vi "Remove Vx from Project.vi"(11 "Project File":path=path "C:/Users/Steve/Documents/LabVIEW/DePuy test rig software new - Playing/DePuy test rig software.lvproj") -> ()   [LabVIEW 2015]
uses:
  Sub VIs/Rename Vx States.ctl
  <vilib>/Utility/file.llb/Write Delimited Spreadsheet (string).vi
  <vilib>/Utility/file.llb/Read Delimited Spreadsheet (string).vi
  <vilib>/LabVIEW Icon API/LabVIEW Icon API.lvlib
panel:
  out "Count":i32
  out "All VIs Count":i32
  in  "Edit ICONs":bool
  out "State":T1
  in  "Delete Originals":bool
  out "Rename Array":path[][](array[path])
  out "All VIs":path[](array[path])
  out "All VI Files":path
  in  "ReLink VIs":bool
  in  "Rename Files in Project":bool
  in  "Revert":bool
  in  "Rename Files":bool
  in  "Load Rename File":bool
  in  "Save Rename File":bool
  out "Rename Files":path
  in  "Read Project":bool
  in  "Stop":bool
  out "Selection Array":T2(array[cluster])
  in  "Ignore Folders":path[](array[path])=[path "C:/Users/Steve/Documents/LabVIEW/DePuy test rig software new - Playing/data", path "C:/Users/Steve/Documents/LabVIEW/DePuy test rig software new - Playing/DLLs", path "C:/Users/Steve/Documents/LabVIEW/DePuy test rig software new - Playing/sub vis/data", path "C:/Users/Steve/Documents/LabVIEW/DePuy test rig software new - Playing/sub vis/data old", path "C:/Users/Steve/Documents/LabVIEW/DePuy test rig software new - Playing/Mathcad Worksheets"]
  # "COMMIT Renamed Files\n    Change Missing to Deleted\n    Change Unknown to Added\n    All should show as Renamed"
  # "Cancel in ICON Editor to Stop"
  # "COMMIT Relinked Files"
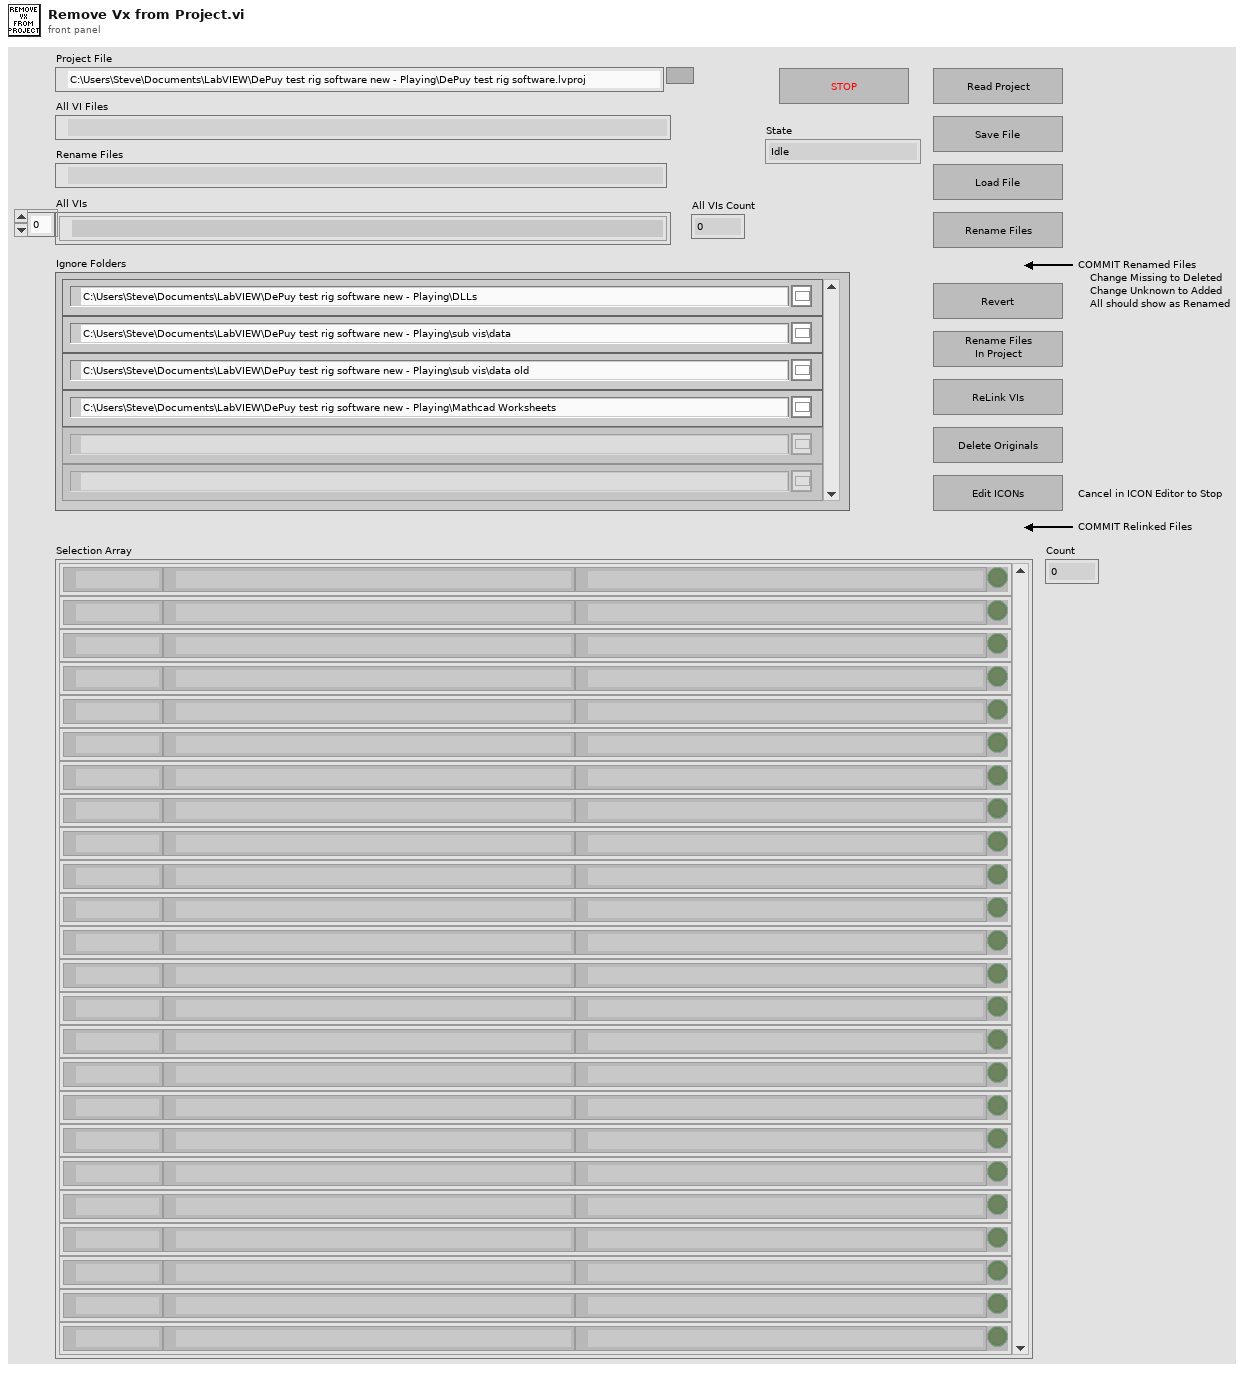
[diagram p1: front panel]
types:
  T1 = typedef "Rename Vx States.ctl" = enum16{"Idle", "Read Project", "Save File", "Load File", "Rename Files", "Revert", "Rename Files in Project", "Delete Originals", "Relink VIs", "Edit ICONs", "Exit"}
  T2 = cluster{"Original":path, "Name":path, "Rename":path, "Change":bool}[]
  T3 = cluster{"Original":path, "Name":path, "Rename":path, "Change":bool}
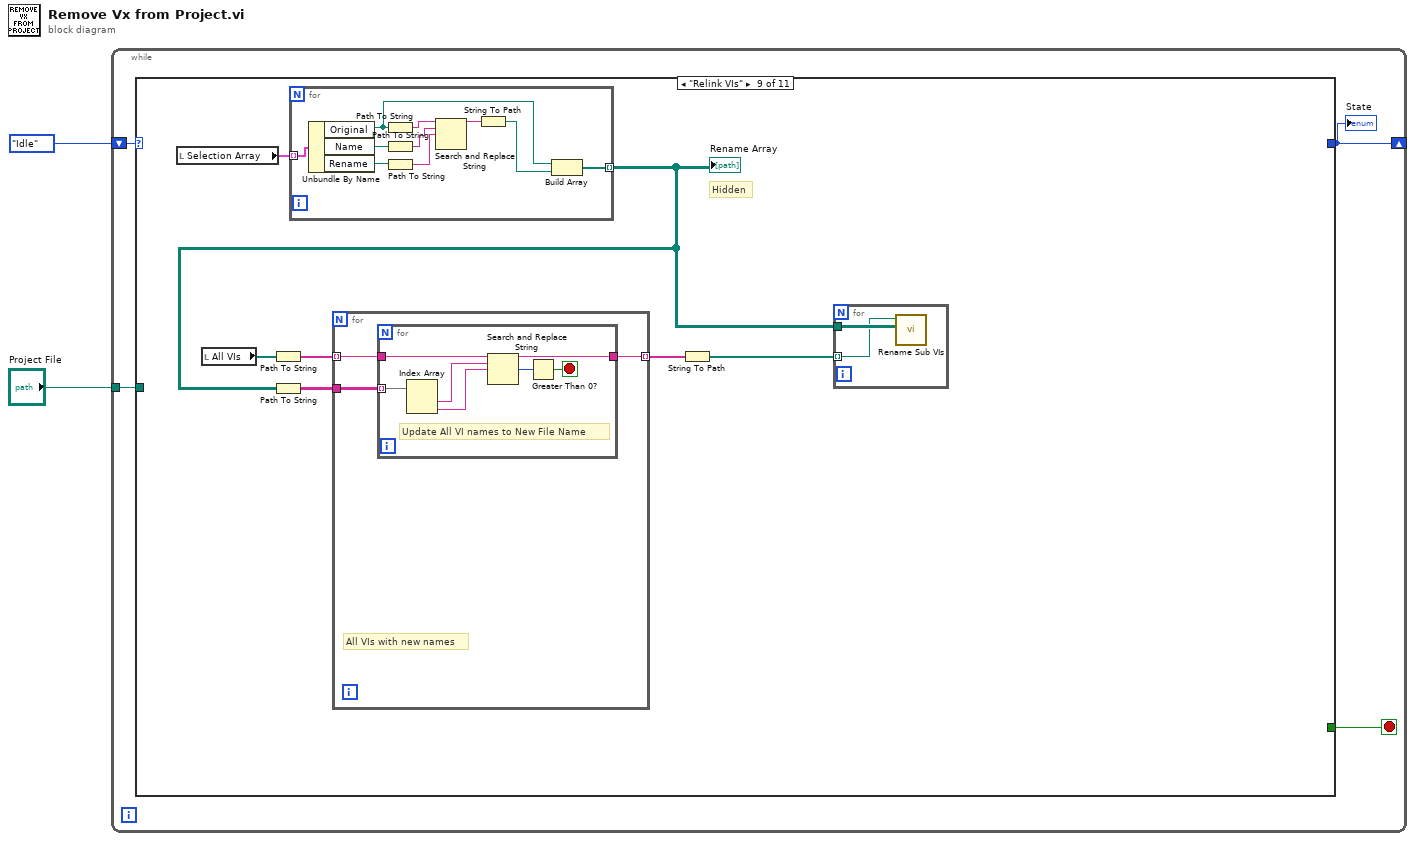
[diagram p0: block diagram]
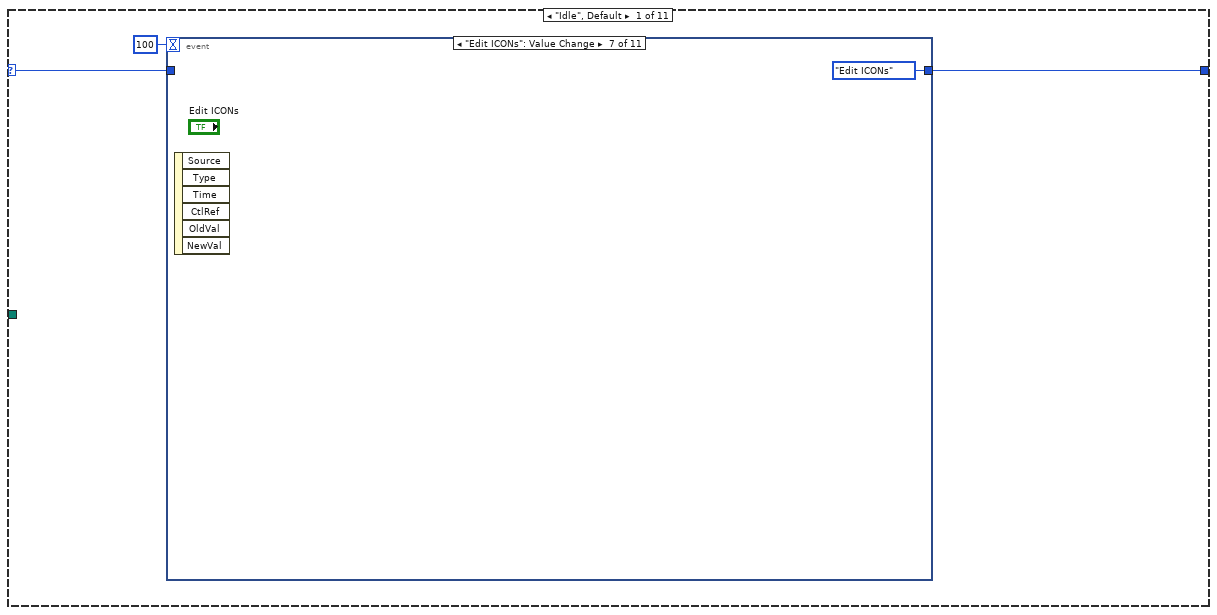
[diagram p2: hidden frame]
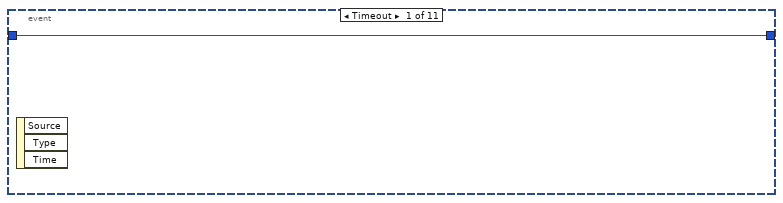
[diagram p3: hidden frame]
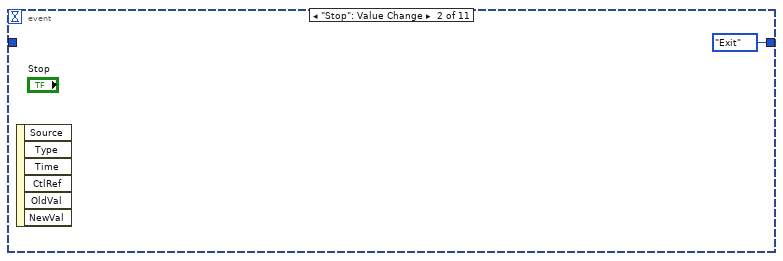
[diagram p4: hidden frame]
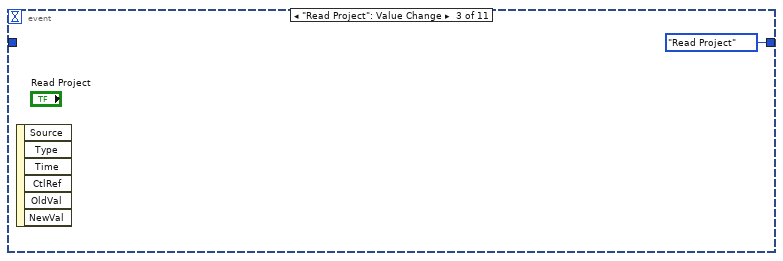
[diagram p5: hidden frame]
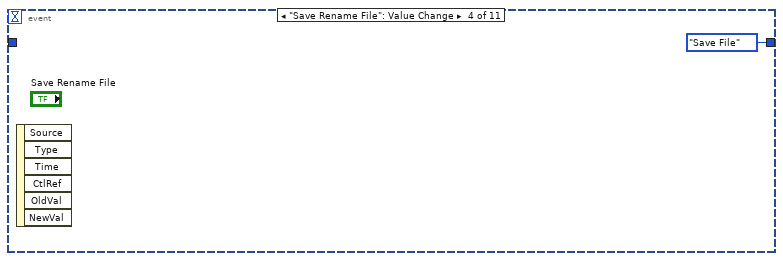
[diagram p6: hidden frame]
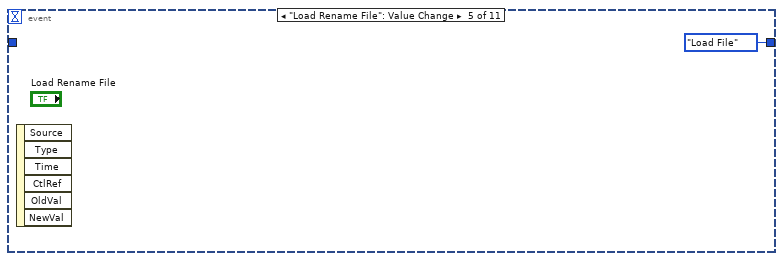
[diagram p7: hidden frame]
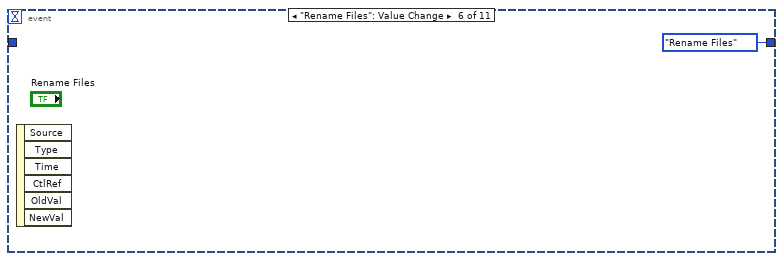
[diagram p8: hidden frame]
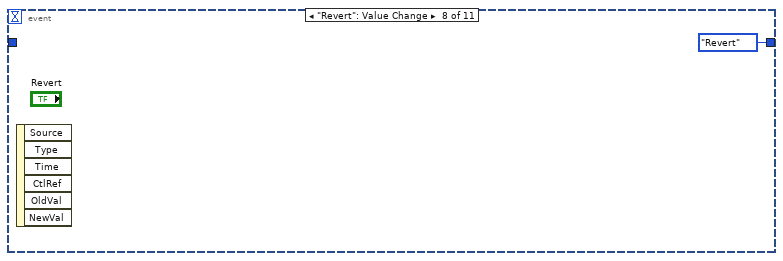
[diagram p9: hidden frame]
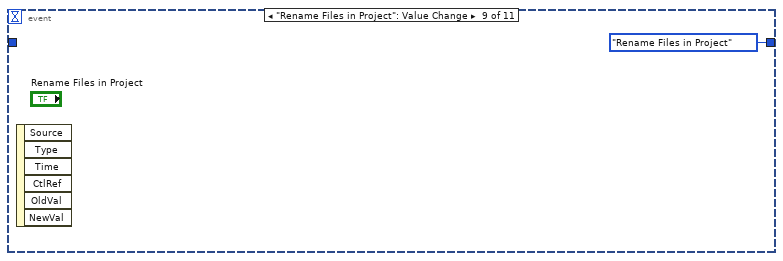
[diagram p10: hidden frame]
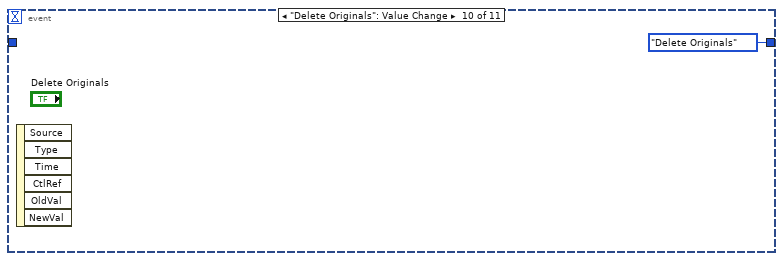
[diagram p11: hidden frame]
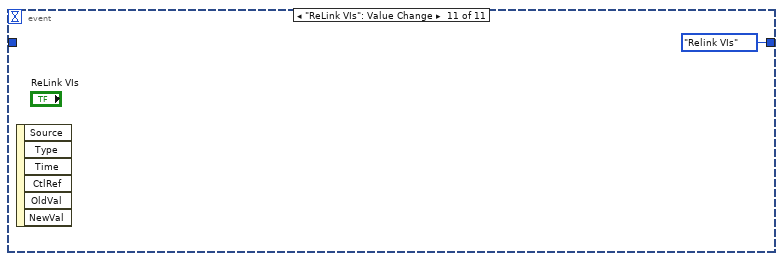
[diagram p12: hidden frame]
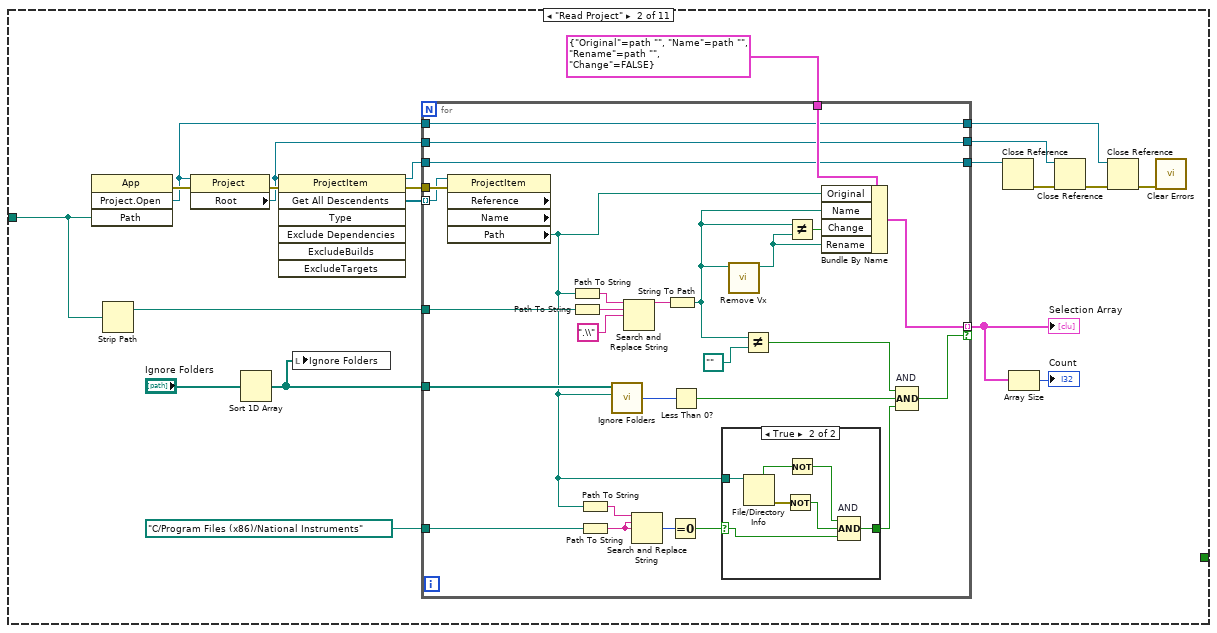
[diagram p13: hidden frame]
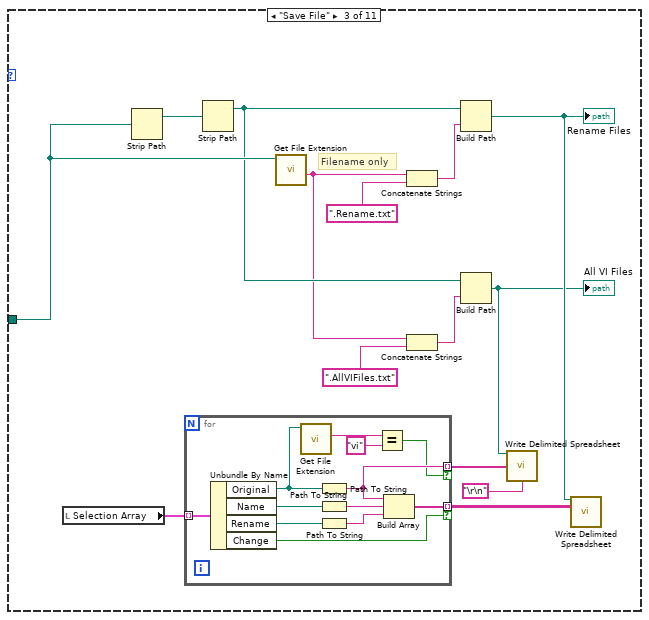
[diagram p15: hidden frame]
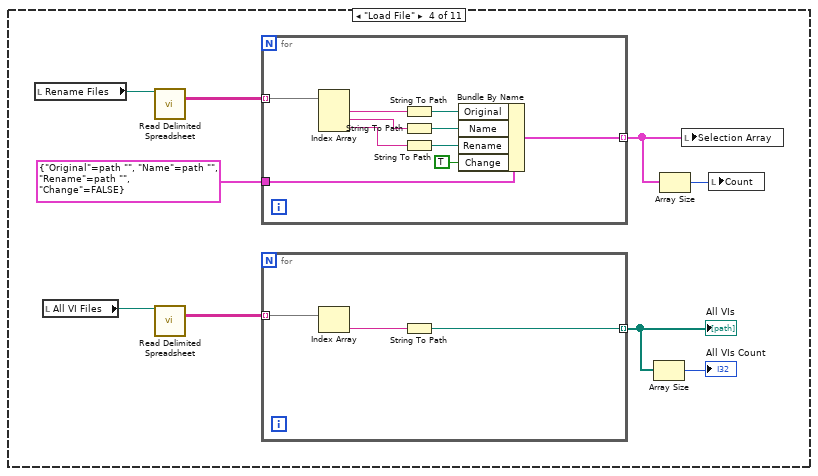
[diagram p16: hidden frame]
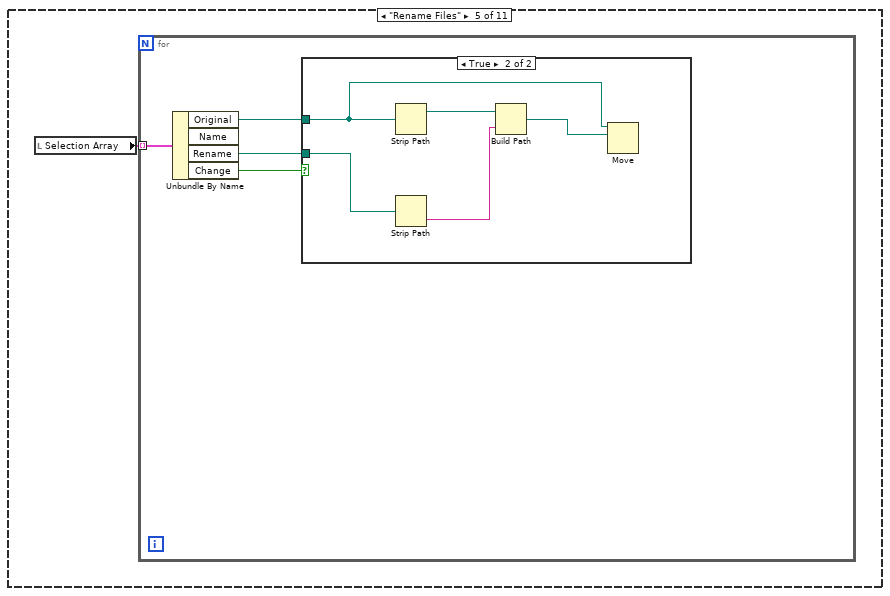
[diagram p17: hidden frame]
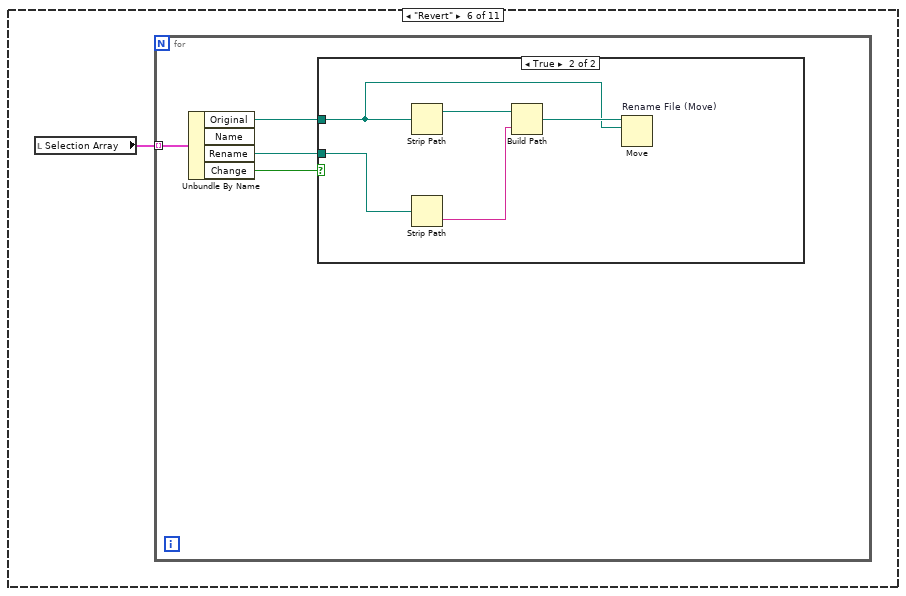
[diagram p19: hidden frame]
diagram:
  n1 = while {
    tunnel: "Project File" -> [w6]
    shift-right: [w5] -> _
    shift-left: Rename_Vx_States."Idle" -> [w4]
    stop <- w3 stop-if-true
    n2 = case shown="\"Relink VIs\"" w4 {
      selector: w4 -> [w7 _ _ _ _ _ _ _ _ _ _]
      tunnel: w6 -> [_ w38 w89 _ _ _ w148 _ _ _ _]
      tunnel: [w8 _ _ _ _ _ _ _ _ _ _] -> w5
      tunnel: [_ _ _ _ _ _ _ _ _ _ TRUE] -> w3
      frame "Idle", Default {
        n3 = event shown="[6] \"Edit ICONs\": Value Change" {
          selector: _ -> [_ _ _ _ _ _ _ _ _ _ _]
          dyn-events: _ -> [_ _ _ _ _ _ _ _ _ _ _]
          timeout: 100 -> [_ _ _ _ _ _ _ _ _ _ _]
          tunnel: [w10 Rename_Vx_States."Exit" Rename_Vx_States."Read Project" Rename_Vx_States."Save File" Rename_Vx_States."Load File" Rename_Vx_States."Rename Files" Rename_Vx_States."Edit ICONs" Rename_Vx_States."Revert" Rename_Vx_States."Rename Files in Project" Rename_Vx_States."Delete Originals" Rename_Vx_States."Relink VIs"] -> w8
          tunnel: w7 -> [w10 _ _ _ _ _ _ _ _ _ _]
          event Timeout {
            n4 = event-data() -> ()  [unwired: 1 in, 3 out]
          }
          event "Stop": Value Change {
            n5 = event-data() -> ()  [unwired: 1 in, 6 out]
          }
          event "Read Project": Value Change {
            n6 = event-data() -> ()  [unwired: 1 in, 6 out]
          }
          event "Save Rename File": Value Change {
            n7 = event-data() -> ()  [unwired: 1 in, 6 out]
          }
          event "Load Rename File": Value Change {
            n8 = event-data() -> ()  [unwired: 1 in, 6 out]
          }
          event "Rename Files": Value Change {
            n9 = event-data() -> ()  [unwired: 1 in, 6 out]
          }
          event "Edit ICONs": Value Change {
            n10 = event-data() -> ()  [unwired: 1 in, 6 out]
          }
          event "Revert": Value Change {
            n11 = event-data() -> ()  [unwired: 1 in, 6 out]
          }
          event "Rename Files in Project": Value Change {
            n12 = event-data() -> ()  [unwired: 1 in, 6 out]
          }
          event "Delete Originals": Value Change {
            n13 = event-data() -> ()  [unwired: 1 in, 6 out]
          }
          event "ReLink VIs": Value Change {
            n14 = event-data() -> ()  [unwired: 1 in, 6 out]
          }
        }
      }
      frame "Read Project" {
        n15 = invoke class="App" method="Project.Open"("Path"=w38) -> (error out=w32:errorcluster, "Project:Open"=w29:refnum<vi>)  [unwired: 3 in, 2 out]
        n16 = Strip Path(path=w38) -> (stripped path=w37:path)  [unwired: 1 out]
        n17 = property class="Project"(reference=w29, error in=w32) -> (error out=w39:errorcluster, "Root"=w30:refnum<vi>)  [unwired: 1 out]
        n18 = Sort 1D Array(array="Ignore Folders") -> (sorted array=w35:path[])
        n19 = invoke class="ProjectItem" method="Get All Descendents"(reference=w30, error in=w39) -> (reference out=w31:refnum<vi>, error out=w40:errorcluster, "All Descendents"=w41:refnum<vi>[])  [unwired: 5 in, 4 out]
        n20 = local write "Ignore Folders"(w35) -> ()
        n21 = for {
          tunnel: w40 -> [w69]
          tunnel: w41 -> [w68] mode=indexing
          tunnel: [w49] -> w22 mode=indexing if=w57
          tunnel: w37 -> [w60]
          tunnel: w35 -> [w58]
          tunnel: path "C:/Program Files (x86)/National Instruments" ("Path") -> [w54]
          tunnel: T3 {"Original"=path "", "Name"=path "", "Rename"=path "", "Change"=FALSE} -> [w48]
          tunnel: [w44] -> w28
          tunnel: w31 -> [w44]
          tunnel: [w43] -> w25
          tunnel: w30 -> [w43]
          tunnel: [w42] -> w24
          tunnel: w29 -> [w42]
          n22 = property class="ProjectItem" props=["Reference", "Name", "Path"](reference=w68, error in=w69) -> ("Path"=w50:path)  [unwired: 4 out]
          n23 = Path To String(path=w50) -> (string=w63:string)
          n24 = Path To String(path=w60) -> (string=w62:string)
          n25 = Path To String(path=w50) -> (string=w65:string)
          n26 = Path To String(path=w54) -> (string=w66:string)
          n27 = call "Ignore Folders.vi"("File"=w50, "Ignore Folders"=w58) -> ("index of element"=w56:i32)  [unwired: 2 in]
          n28 = Search and Replace String(input string=w63, search string=w62, replace string=".\\" ("replace string (\"\")")) -> (result string=w61:string)  [unwired: 5 in, 3 out]
          n29 = Search and Replace String(input string=w65, search string=w66, replace string=w66) -> (number of replacements=w64:i32)  [unwired: 5 in, 3 out]
          n30 = String To Path(string=w61) -> (path=w46:path)
          n31 = Equal To 0?(x=w64) -> (x = 0?=w52:bool)
          n32 = Less Than 0?(x=w56) -> (x < 0?=w53:bool)
          n33 = case shown="True" w52 {
            selector: w52 -> [w70 w73]
            tunnel: [w70 w74] -> w51
            tunnel: w50 -> [_ w77]
            frame False {
            }
            frame True {
              n34 = File/Directory Info(path=w77) -> (directory=w76:bool, error out=w75:errorcluster)  [unwired: 1 in, 5 out]
              n35 = Not(x=w75) -> (.not. x?=w72:bool)
              n36 = Not(x=w76) -> (.not. x?=w71:bool)
              n37 = Compound Arithmetic op=AND "AND"(w71, w72, w73) -> (w74:bool)
            }
          }
          n38 = call "Remove Vx.vi"("Path in"=w46) -> ("Path out"=w45:path)  [unwired: 10 in]
          n39 = Not Equal?(x=w46, y=path "" ("Path")) -> (x != y?=w55:bool)
          n40 = Not Equal?(x=w46, y=w45) -> (x != y?=w47:bool)
          n41 = Bundle By Name(cluster=w48, "Original"=w50, "Name"=w46, "Change"=w47, "Rename"=w45) -> (w49:T3)
          n42 = Compound Arithmetic op=AND "AND"(w55, w53, w51) -> (w57:bool)
        }
        "Selection Array" <- w22
        n43 = Close Reference(reference=w28) -> (error out=w27:errorcluster)  [unwired: 1 in]
        n44 = Array Size(array=w22) -> (size(s)=→"Count":i32)
        n45 = Close Reference(reference=w25, error in (no error)=w27) -> (error out=w26:errorcluster)
        n46 = Close Reference(reference=w24, error in (no error)=w26) -> (error out=w23:errorcluster)
        n47 = call <vilib>:"Clear Errors.vi"("error in (no error)"=w23) -> ()  [unwired: 5 in, 2 out]
      }
      frame "Save File" {
        # "Filename only"
        n48 = local read "Selection Array"() -> (w91:T2)
        n49 = Strip Path(path=w89) -> (stripped path=w90:path)  [unwired: 1 out]
        n50 = for {
          tunnel: w91 -> [w103] mode=indexing
          tunnel: [w98] -> w81 mode=indexing if=w97
          tunnel: [w96] -> w80 mode=indexing if=w92
          n51 = Unbundle By Name(w103) -> ("Original"=w95:path, "Name"=w101:path, "Rename"=w102:path, "Change"=w97:bool)
          n52 = call <vilib>:"Get File Extension.vi"("file"=w95) -> ("lowercase file extension"=w94:string)  [unwired: 6 in, 4 out]
          n53 = Path To String(path=w95) -> (string=w96:string)
          n54 = Path To String(path=w101) -> (string=w100:string)
          n55 = Path To String(path=w102) -> (string=w99:string)
          n56 = Equal?(x=w94, y="vi") -> (x = y?=w92:bool)
          n57 = Build Array(w96, w100, w99) -> (w98:string[])
        }
        n58 = Strip Path(path=w90) -> (stripped path=w83:path)  [unwired: 1 out]
        n59 = call <vilib>:"Get File Extension.vi"("file"=w89) -> ("filename without extension"=w82:string)  [unwired: 6 in, 4 out]
        n60 = Concatenate Strings(w82, ".Rename.txt" ("string")) -> (w87:string)
        n61 = Concatenate Strings(w82, ".AllVIFiles.txt" ("string")) -> (w85:string)
        n62 = Build Path(base path=w83, name or relative path=w87) -> (appended path=w86:path)
        "Rename Files" <- w86
        n63 = Build Path(base path=w83, name or relative path=w85) -> (appended path=w79:path)
        "All VI Files" <- w79
        n64 = call-poly <vilib>:"Write Delimited Spreadsheet.vi"("file path (dialog if empty)"=w79, "1D data"=w80, "delimiter (\\t)"="\r\n") -> ()  [unwired: 11 in, 2 out]
        n65 = call-poly <vilib>:"Write Delimited Spreadsheet.vi"("file path (dialog if empty)"=w86, "2D data"=w81) -> ()  [unwired: 12 in, 2 out]
      }
      frame "Load File" {
        n66 = local read "Rename Files"() -> (w112:path)
        n67 = local read "All VI Files"() -> (w109:path)
        n68 = call-poly <vilib>:"Read Delimited Spreadsheet.vi"("file path (dialog if empty)"=w112) -> ("all rows"=w111:string[][])  [unwired: 9 in, 5 out]
        n69 = call-poly <vilib>:"Read Delimited Spreadsheet.vi"("file path (dialog if empty)"=w109) -> ("all rows"=w108:string[][])  [unwired: 9 in, 5 out]
        n70 = for {
          tunnel: w111 -> [w123] mode=indexing
          tunnel: T3 {"Original"=path "", "Name"=path "", "Rename"=path "", "Change"=FALSE} -> [w125]
          tunnel: [w116] -> w105 mode=indexing
          n71 = Index Array(array=w123) -> (element #1=w122:string, element #2=w118:string, element #3=w117:string)  [unwired: 3 in]
          n72 = String To Path(string=w122) -> (path=w121:path)
          n73 = String To Path(string=w118) -> (path=w119:path)
          n74 = String To Path(string=w117) -> (path=w120:path)
          n75 = Bundle By Name(cluster=w125, "Original"=w121, "Name"=w119, "Rename"=w120, "Change"=TRUE) -> (w116:T3)
        }
        n76 = for {
          tunnel: w108 -> [w114] mode=indexing
          tunnel: [w115] -> w107 mode=indexing
          n77 = Index Array(array=w114) -> (element=w113:string)  [unwired: 1 in]
          n78 = String To Path(string=w113) -> (path=w115:path)
        }
        "All VIs" <- w107
        n79 = Array Size(array=w107) -> (size(s)=→"All VIs Count":i32)
        n80 = Array Size(array=w105) -> (size(s)=w104:i32)
        n81 = local write "Selection Array"(w105) -> ()
        n82 = local write "Count"(w104) -> ()
      }
      frame "Rename Files" {
        n83 = local read "Selection Array"() -> (w126:T2)
        n84 = for {
          tunnel: w126 -> [w130] mode=indexing
          n85 = Unbundle By Name(w130) -> ("Original"=w128:path, "Rename"=w129:path, "Change"=w127:bool)  [unwired: 1 out]
          n86 = case shown="True" w127 {
            tunnel: w129 -> [_ w135]
            tunnel: w128 -> [_ w132]
            frame False {
            }
            frame True {
              n87 = Strip Path(path=w132) -> (stripped path=w134:path)  [unwired: 1 out]
              n88 = Strip Path(path=w135) -> (name=w133:string)  [unwired: 1 out]
              n89 = Build Path(base path=w134, name or relative path=w133) -> (appended path=w131:path)
              n90 = Move(source path=w132, 10:w131) -> ()  [unwired: 3 in, 3 out]
            }
          }
        }
      }
      frame "Revert" {
        n91 = local read "Selection Array"() -> (w136:T2)
        n92 = for {
          tunnel: w136 -> [w140] mode=indexing
          n93 = Unbundle By Name(w140) -> ("Original"=w138:path, "Rename"=w139:path, "Change"=w137:bool)  [unwired: 1 out]
          n94 = case shown="True" w137 {
            tunnel: w139 -> [_ w145]
            tunnel: w138 -> [_ w141]
            frame False {
            }
            frame True {
              n95 = Strip Path(path=w141) -> (stripped path=w144:path)  [unwired: 1 out]
              n96 = Strip Path(path=w145) -> (name=w143:string)  [unwired: 1 out]
              n97 = Build Path(base path=w144, name or relative path=w143) -> (appended path=w142:path)
              n98 = Move "Rename File (Move)"(source path=w142, 10:w141) -> ()  [unwired: 3 in, 3 out]
            }
          }
        }
      }
      frame "Rename Files in Project" {
        n99 = invoke class="App" method="Project.Open"("Path"=w148) -> (error out=w154:errorcluster, "Project:Open"=w147:refnum<vi>)  [unwired: 3 in, 2 out]
        n100 = invoke class="Project" method="Open Window"(reference=w147) -> (reference out=w146:refnum<vi>)  [unwired: 2 in, 2 out]
        n101 = property class="Project"(reference=w146, error in=w154) -> (reference out=w150:refnum<vi>, error out=w158:errorcluster, "Root"=w159:refnum<vi>)
        n102 = local read "Ignore Folders"() -> (w157:path[])
        n103 = local read "Selection Array"() -> (w151:T2)
        n104 = invoke class="ProjectItem" method="Get All Descendents"(reference=w159, error in=w158) -> (reference out=w152:refnum<vi>, error out=w160:errorcluster, "All Descendents"=w161:refnum<vi>[])  [unwired: 5 in, 4 out]
        n105 = for {
          tunnel: w160 -> [w179]
          tunnel: w161 -> [w178] mode=indexing
          tunnel: w157 -> [w174]
          tunnel: path "C:/Program Files (x86)/National Instruments" ("Path") -> [w172]
          tunnel: T3 {"Original"=path "", "Name"=path "", "Rename"=path "", "Change"=FALSE} -> [_]
          tunnel: [w168] -> w153
          tunnel: w152 -> [w168]
          tunnel: w151 -> [w167]
          tunnel: [w162] -> w149
          tunnel: w150 -> [w162]
          n106 = property class="ProjectItem" props=["Reference", "Name", "Path"](reference=w178, error in=w179) -> (error out=w164:errorcluster, "Reference"=w165:refnum<vi>, "Path"=w166:path)  [unwired: 2 out]
          n107 = Path To String(path=w166) -> (string=w176:string)
          n108 = Path To String(path=w172) -> (string=w177:string)
          n109 = call "Ignore Folders.vi"("File"=w166, "Ignore Folders"=w174) -> ("index of element"=w173:i32)  [unwired: 2 in]
          n110 = Search and Replace String(input string=w176, search string=w177, replace string=w177) -> (number of replacements=w175:i32)  [unwired: 5 in, 3 out]
          n111 = Equal To 0?(x=w175) -> (x = 0?=w170:bool)
          n112 = Less Than 0?(x=w173) -> (x < 0?=w171:bool)
          n113 = case shown="True" w170 {
            selector: w170 -> [w204 w207]
            tunnel: [w204 w208] -> w169
            tunnel: w166 -> [_ w211]
            frame False {
            }
            frame True {
              n114 = File/Directory Info(path=w211) -> (directory=w210:bool, error out=w209:errorcluster)  [unwired: 1 in, 5 out]
              n115 = Not(x=w209) -> (.not. x?=w206:bool)
              n116 = Not(x=w210) -> (.not. x?=w205:bool)
              n117 = Compound Arithmetic op=AND "AND"(w205, w206, w207) -> (w208:bool)
            }
          }
          n118 = And(x=w171, y=w169) -> (x .and. y?=w163:bool)
          n119 = case shown="True" w163 {
            tunnel: w167 -> [_ w186]
            tunnel: w166 -> [_ w185]
            tunnel: w165 -> [_ w181]
            tunnel: w164 -> [_ w180]
            frame False {
            }
            frame True {
              n120 = for {
                tunnel: w186 -> [w203] mode=indexing
                tunnel: w185 -> [w198]
                tunnel: [w199] -> w184
                tunnel: [w198] -> w183
                tunnel: [w197] -> w182
                stop <- w200 stop-if-true
                n121 = Unbundle By Name(w203) -> ("Original"=w202:path, "Rename"=w197:path, "Change"=w201:bool)  [unwired: 1 out]
                n122 = Equal?(x=w198, y=w202) -> (x = y?=w200:bool)
                n123 = And(x=w200, y=w201) -> (x .and. y?=w199:bool)
              }
              n124 = case shown="True" w184 {
                tunnel: w182 -> [_ w194]
                tunnel: w183 -> [_ w193]
                tunnel: w181 -> [_ w191]
                tunnel: w180 -> [_ w187]
                frame False {
                }
                frame True {
                  w190 = FALSE ("Save a Copy")
                  n125 = Strip Path(path=w193) -> (stripped path=w196:path)  [unwired: 1 out]
                  n126 = Strip Path(path=w194) -> (name=w195:string)  [unwired: 1 out]
                  n127 = Build Path(base path=w196, name or relative path=w195) -> (appended path=w192:path)
                  n128 = invoke class="VI" method="Save.Instrument"(reference=w191, error in=w187, "Path to saved file"=w192, "Save a Copy"=w190, "Without Diagram"=w190) -> (reference out=w188:refnum<vi>, error out=w189:errorcluster)  [unwired: 1 in, 4 out]
                  n129 = Close Reference(reference=w188, error in (no error)=w189) -> ()  [unwired: 1 out]
                }
              }
            }
          }
        }
        n130 = invoke class="Project" method="Save"(reference=w149, "Path"=w148) -> ()  [unwired: 2 in, 4 out]
        n131 = Close Reference(reference=w153) -> ()  [unwired: 1 in, 1 out]
      }
      frame "Delete Originals" {
        n132 = local read "Selection Array"() -> (w212:T2)
        n133 = for {
          tunnel: w212 -> [w214] mode=indexing
          n134 = Unbundle By Name(w214) -> ("Original"=w213:path)
          n135 = Delete(path (use dialog)=w213) -> ()  [unwired: 4 in, 3 out]
        }
      }
      frame "Relink VIs" {
        # "Hidden"
        n136 = local read "Selection Array"() -> (w221:T2)
        n137 = local read "All VIs"() -> (w220:path[])
        n138 = Path To String(path=w220) -> (string=w219:string[])
        n139 = for {
          tunnel: w221 -> [w241] mode=indexing
          tunnel: [w240] -> w218 mode=indexing
          n140 = Unbundle By Name(w241) -> ("Original"=w232:path, "Name"=w238:path, "Rename"=w239:path)
          n141 = Path To String(path=w232) -> (string=w237:string)
          n142 = Path To String(path=w238) -> (string=w236:string)
          n143 = Path To String(path=w239) -> (string=w235:string)
          n144 = Search and Replace String(input string=w237, search string=w236, replace string=w235) -> (result string=w234:string)  [unwired: 5 in, 3 out]
          n145 = String To Path(string=w234) -> (path=w233:path)
          n146 = Build Array(w232, w233) -> (w240:path[])
        }
        "Rename Array" <- w218
        n147 = Path To String(path=w218) -> (string=w217:string[][])
        n148 = for {
          tunnel: w217 -> [w224]
          tunnel: w219 -> [w223] mode=indexing
          tunnel: [w222] -> w216 mode=indexing
          # "All VIs with new names"
          n149 = for {
            tunnel: w224 -> [w231] mode=indexing
            tunnel: w223 -> [w230]
            tunnel: [w225] -> w222
            stop <- w226 stop-if-true
            # "Update All VI names to New File Name"
            n150 = Index Array(array=w231) -> (element #1=w229:string, element #2=w228:string)  [unwired: 2 in]
            n151 = Search and Replace String(input string=w230, search string=w229, replace string=w228) -> (result string=w225:string, number of replacements=w227:i32)  [unwired: 5 in, 2 out]
            n152 = Greater Than 0?(x=w227) -> (x > 0?=w226:bool)
          }
        }
        n153 = String To Path(string=w216) -> (path=w215:path[])
        n154 = for {
          tunnel: w218 -> [w243]
          tunnel: w215 -> [w242] mode=indexing
          n155 = call "Rename Sub VIs.vi"("Rename Array"=w243, "vi path"=w242) -> ()  [unwired: 9 in, 1 out]
        }
      }
      frame "Edit ICONs" {
        n156 = local read "Selection Array"() -> (w250:T2)
        n157 = local read "All VIs"() -> (w245:path[])
        n158 = Path To String(path=w245) -> (string=w249:string[])
        n159 = for {
          tunnel: w250 -> [w270] mode=indexing
          tunnel: [w269] -> w246 mode=indexing
          n160 = Unbundle By Name(w270) -> ("Original"=w261:path, "Name"=w267:path, "Rename"=w268:path)
          n161 = Path To String(path=w261) -> (string=w266:string)
          n162 = Path To String(path=w267) -> (string=w265:string)
          n163 = Path To String(path=w268) -> (string=w264:string)
          n164 = Search and Replace String(input string=w266, search string=w265, replace string=w264) -> (result string=w263:string)  [unwired: 5 in, 3 out]
          n165 = String To Path(string=w263) -> (path=w262:path)
          n166 = Build Array(w261, w262) -> (w269:path[])
        }
        n167 = Path To String(path=w246) -> (string=w248:string[][])
        n168 = for {
          tunnel: w248 -> [w253]
          tunnel: w249 -> [w252] mode=indexing
          tunnel: [w251] -> w247 mode=indexing
          # "All VIs with new names"
          n169 = for {
            tunnel: w253 -> [w260] mode=indexing
            tunnel: w252 -> [w259]
            tunnel: [w254] -> w251
            stop <- w255 stop-if-true
            # "Update All VI names to New File Name"
            n170 = Index Array(array=w260) -> (element #1=w258:string, element #2=w257:string)  [unwired: 2 in]
            n171 = Search and Replace String(input string=w259, search string=w258, replace string=w257) -> (result string=w254:string, number of replacements=w256:i32)  [unwired: 5 in, 2 out]
            n172 = Greater Than 0?(x=w256) -> (x > 0?=w255:bool)
          }
        }
        n173 = String To Path(string=w247) -> (path=w244:path[])
        n174 = local write "Rename Array"(w246) -> ()
        n175 = for {
          tunnel: w244 -> [w280] mode=indexing
          stop <- w271 stop-if-true
          n176 = Open VI Reference(vi path=w280) -> (vi reference=w275:refnum<vi>, error out=w272:errorcluster)  [unwired: 5 in]
          n177 = call <vilib>:"Get VI Icon.vi"("error in (no error)"=w272, "VI Refnum in"=w275) -> ("error out"=w279:errorcluster, "Icon"=w278:refnum<class "Icon.lvclass">)  [unwired: 7 in, 1 out]
          n178 = call <vilib>:"Launch Icon Editor.vi"("error in (no error)"=w279, "Icon in"=w278) -> ("error out"=w277:errorcluster, "Icon out"=w276:refnum<class "Icon.lvclass">, "Canceled?"=w271:bool)  [unwired: 7 in]
          n179 = call <vilib>:"Set VI Icon.vi"("error in (no error)"=w277, "Icon"=w276, "VI Refnum in"=w275) -> ("error out"=w273:errorcluster, "VI Refnum out"=w274:refnum<vi>)  [unwired: 7 in]
          n180 = case shown="False" w271 {
            tunnel: w274 -> [w282 _]
            tunnel: w273 -> [w281 _]
            frame False {
              n181 = invoke class="VI" method="Save.Instrument"(reference=w282, error in=w281) -> ()  [unwired: 4 in, 6 out]
            }
            frame True {
            }
          }
        }
      }
      frame "Exit" {
      }
    }
    "State" <- w5
  }
